vi "Add Property.vi"(7 "MsgSerializer":refnum<class "MsgSerializer.lvclass">, 10 "Property":variant, 11 "Test Suite in":refnum<class "Test Suite.lvclass">) -> (3 "Test Suite out":refnum<class "Test Suite.lvclass">)   [LabVIEW 2013, in "JUnit Conversion.lvlib"]
uses:
  JUnit Conversion.lvlib
  <vilib>/addons/_JKI Toolkits/Caraya/classes/MsgSerializer/MsgSerializer.lvclass
  <vilib>/PNR/JUnit XML/JUnit XML/Test Suite/Test Suite.lvclass
  <vilib>/PNR/JUnit XML/JUnit XML/Property/Property.lvclass
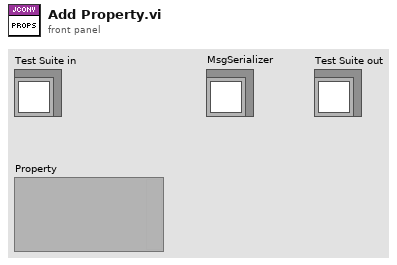
[diagram p1: front panel]
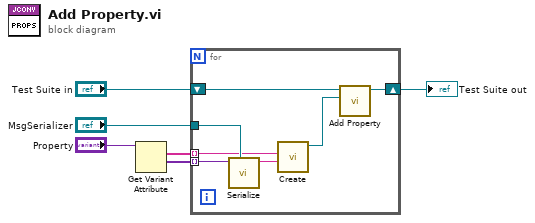
[diagram p0: block diagram]
diagram:
  n1 = Get Variant Attribute(Variant="Property") -> (names=w6:string[], values=w5:variant[])  [unwired: 3 in, 2 out]
  n2 = for {
    tunnel: w6 -> [w10] mode=indexing
    tunnel: w5 -> [w13] mode=indexing
    tunnel: "MsgSerializer" -> [w12]
    shift-right: [w8] -> w2
    shift-left: "Test Suite in" -> [w7]
    n3 = call-dynamic "Serialize.vi"("MsgSerializer"=w12, "Value"=w13) -> ("Serialized Message"=w11:string)  [unwired: 8 in, 1 out]
    n4 = call <vilib>:"Create.vi"("Value"=w11, "Name"=w10) -> ("Property"=w9:refnum<class "Property.lvclass">)  [unwired: 8 in, 1 out]
    n5 = call <vilib>:"Add Property.vi"("Property"=w9, "Test Suite in"=w7) -> ("Test Suite out"=w8:refnum<class "Test Suite.lvclass">)  [unwired: 8 in, 1 out]
  }
  "Test Suite out" <- w2
